vi "(BASVR) Configure AVS.vi"(6 "error in (no error)":errorcluster, 11 "input cluster":T2) -> (0 "Chosen Channel":i32, 1 "Channel Start Time":timestamp, 2 "Chosen Channel Index":i32, 3 "Configuration Cluster":T1, 4 "error out":errorcluster)   [LabVIEW 2023]
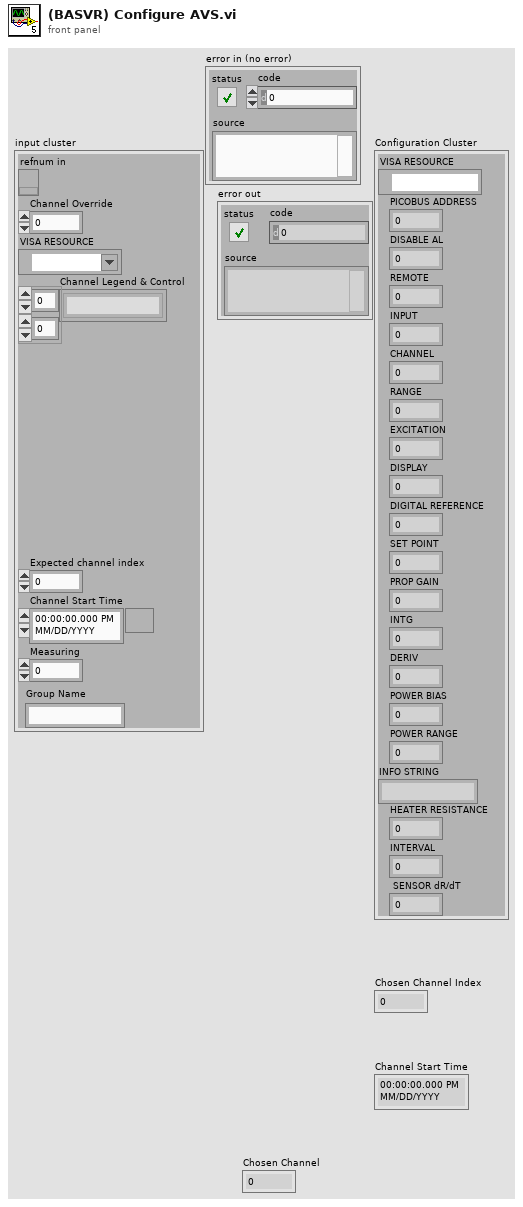
[diagram p1: front panel]
types:
  T1 = cluster{"VISA RESOURCE":refnum<visa-resource-name>, "PICOBUS ADDRESS":u8, "DISABLE AL":u8, "REMOTE":u8, "INPUT":u8, "CHANNEL":u8, "RANGE":u8, "EXCITATION":u8, "DISPLAY":u8, "DIGITAL REFERENCE":u16, "SET POINT":dbl, "PROP GAIN":u8, "INTG":u8, "DERIV":u8, "POWER BIAS":u8, "POWER RANGE":u8, "INFO STRING":string, "HEATER RESISTANCE":dbl, "INTERVAL":u8, " SENSOR dR/dT":u8}
  T2 = cluster{"refnum in":refnum<k34>, "Channel Override":u16, "VISA RESOURCE":refnum<visa-resource-name>, "Channel Legend & Control":string[][], "Expected channel index":i32, "Channel Start Time":timestamp, "Measuring":i32, "Group Name":string}
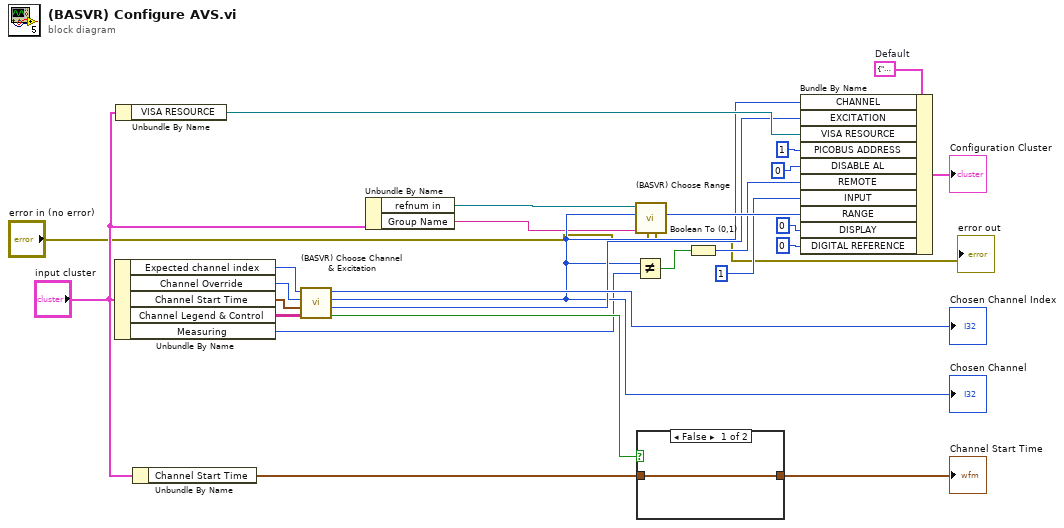
[diagram p0: block diagram]
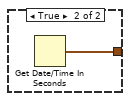
[diagram p2: hidden frame]
diagram:
  w9 = T1 {"VISA RESOURCE"="COM5", "PICOBUS ADDRESS"=1, "DISABLE AL"=0, "REMOTE"=1, "INPUT"=1, "CHANNEL"=0, "RANGE"=5, "EXCITATION"=4, "DISPLAY"=0, "DIGITAL REFERENCE"=0, "SET POINT"=0.0, "PROP GAIN"=0, "INTG"=0, "DERIV"=0, "POWER BIAS"=0, "POWER RANGE"=0, "INFO STRING"="", "HEATER RESISTANCE"=0.0, "INTERVAL"=0, " SENSOR dR/dT"=0}  # Default
  n1 = Unbundle By Name("input cluster") -> ("Expected channel index"=w24:i32, "Channel Override"=w25:u16, "Channel Start Time"=w26:timestamp, "Channel Legend & Control"=w27:string[][], "Measuring"=w4:i32)
  n2 = Unbundle By Name("input cluster") -> ("VISA RESOURCE"=w22:refnum<visa-resource-name>)
  n3 = Unbundle By Name("input cluster") -> ("Channel Start Time"=w7:timestamp)
  n4 = call "(BASVR) Choose Channel & Excitation.vi"("Channel Legend & Control"=w27, "Channel Start TIme"=w26, "Channel Override"=w25, "Expected Channel Index"=w24) -> ("Channel Changed?"=w18:bool, "Chosen Excitaiton"=w6:u8, "Chosen Channel"=w5:i32, "Chosen Channel Index"=→"Chosen Channel Index":i32)  [unwired: 4 in]
  "Chosen Channel" <- w5
  n5 = Unbundle By Name("input cluster") -> ("refnum in"=w23:refnum<k34>, "Group Name"=w3:string)
  n6 = Not Equal?(x=w5, y=w4) -> (x != y?=w21:bool)
  n7 = call "(BASVR) Choose Range.vi"("error in (no error)"="error in (no error)", "Group Name"=w3, "Chosen Channel"=w5, "tdms ref"=w23) -> ("Chosen Range"=w17:u8, "error out"=→"error out":errorcluster)  [unwired: 6 in]
  n8 = case shown="False" w18 {
    tunnel: [w28 w29] -> w19
    tunnel: w7 -> [w28 _]
    frame False {
    }
    frame True {
      n9 = Get Date/Time In Seconds() -> (seconds since 1Jan1904=w29:timestamp)
    }
  }
  "Channel Start Time" <- w19
  n10 = Boolean To (0,1)(Boolean=w21) -> (0, 1=w16:i16)
  n11 = Bundle By Name(cluster=w9, "CHANNEL"=w5, "EXCITATION"=w6, "VISA RESOURCE"=w22, "PICOBUS ADDRESS"=u8 1, "DISABLE AL"=u8 0, "REMOTE"=w16, "INPUT"=u8 1, "RANGE"=w17, "DISPLAY"=u8 0, "DIGITAL REFERENCE"=u16 0) -> (→"Configuration Cluster":T1)
